vi "s-lab第3章 字符串数据1-13.vi"() -> ()   [LabVIEW 2013]
panel:
  out "密码形式显示":string(combo)
  out "字符串正常显示":string
  in  "组合框":string(combo)
  out "字符串 7":string
  out "布尔":bool
  in  "假字符串":string
  in  "真字符串":string
  in  "字符串 6":string
  out "位置":dbl
  in  "数组":string[](array[string])
  in  "欲查找字符串":string
  out "系统时间戳":string
  out "字符串 5":string
  in  "要更正的字符串":string
  in  "要查找的字符串":string
  in  "源字符串":string
  in  "插入位置":dbl
  out "插入后的字符串":string
  in  "要插入的字符串":string
  in  "原字符串":string
  in  "截取字符串长度 2":dbl
  in  "偏移量 2":dbl
  out "被替换的字符串":string
  in  "替换字符串":string
  out "替换结果":string
  in  "原有字符串":string
  out "大写字符串":string
  in  "小写字符串":string
  in  "截取字符串长度":dbl
  in  "偏移量":dbl
  out "子字符串":string
  in  "字符串 4":string
  out "连接后的字符串":string
  in  "字符串 3":string
  in  "字符串 2":string
  out "数值":dbl
  in  "字符串":string
  # "字符串的长度"
  # "例 1"
  # "例 8"
  # "例 9"
  # "例 2"
  # "例 10"
  # "例 3"
  # "例 11"
  # "例 4"
  # "例 5"
  # "例 12"
  # "例 6"
  # "例 13"
  # "例 7"
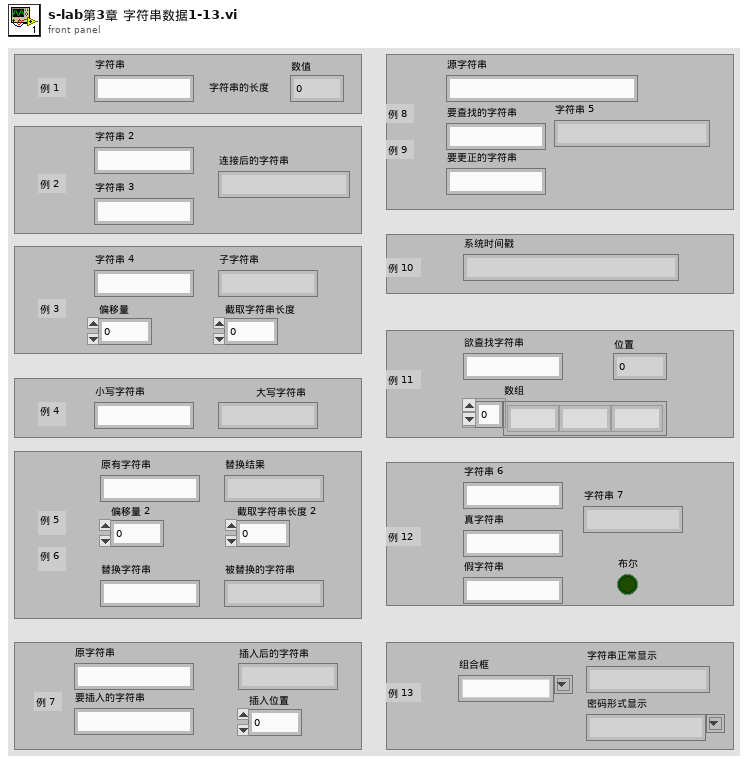
[diagram p1: front panel]
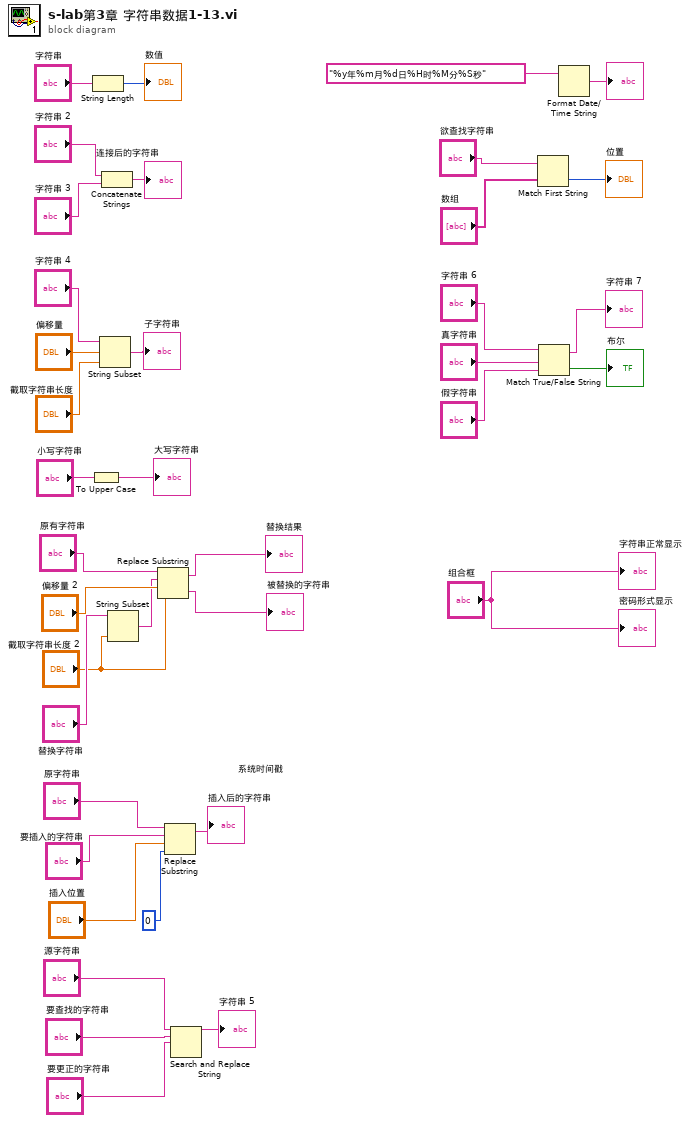
[diagram p0: block diagram]
diagram:
  n1 = To Upper Case(1:"小写字符串") -> (0:→"大写字符串":string)
  n2 = String Length(string="字符串") -> (length=→"数值":i32)
  n3 = String Subset(string="字符串 4", offset (0)="偏移量", length (rest)="截取字符串长度") -> (substring=→"子字符串":string)
  n4 = Concatenate Strings("字符串 2", "字符串 3") -> (→"连接后的字符串":string)
  n5 = String Subset(string="替换字符串", length (rest)="截取字符串长度 2") -> (substring=w24:string)  [unwired: 1 in]
  n6 = Replace Substring(2:"截取字符串长度 2", 3:"偏移量 2", 4:w24, 5:"原有字符串") -> (0:→"被替换的字符串":string, 1:→"替换结果":string)
  n7 = Replace Substring(2:0, 3:"插入位置", 4:"要插入的字符串", 5:"原字符串") -> (1:→"插入后的字符串":string)  [unwired: 1 out]
  n8 = Search and Replace String(input string="源字符串", search string="要查找的字符串", replace string="要更正的字符串") -> (result string=→"字符串 5":string)  [unwired: 5 in, 3 out]
  n9 = Match First String(2:"数组", 3:"欲查找字符串") -> (0:→"位置":i32)  [unwired: 1 out]
  n10 = Match True/False String(2:"假字符串", 3:"真字符串", 4:"字符串 6") -> (0:→"布尔":bool, 1:→"字符串 7":string)
  n11 = Format Date/Time String(time format string (%c)="%y年%m月%d日%H时%M分%S秒") -> (date/time string=→"系统时间戳":string)  [unwired: 2 in]
  "字符串正常显示" <- "组合框"
  "密码形式显示" <- "组合框"
